vi "Next Post Processor Name.vi"(7 "Ack Result":refnum<class "Acquired Result.lvclass">, 8 "error in (no error)":errorcluster, 11 "Monitor-Pulse in":refnum<class "Batch Processor.lvclass">) -> (0 "error out":errorcluster, 1 "Complete":bool, 2 "Post processor name":string, 3 "Monitor-Pulse out":refnum<class "Batch Processor.lvclass">, 5 "Ack Result out":refnum<class "Acquired Result.lvclass">)   [LabVIEW 2020, in "Batch Processor.lvclass"]
uses:
  Batch Processor.lvclass
  C:/GitHub/LabActor/Worker/Worker.lvclass
  C:/Program Files/National Instruments/LabVIEW 2020/vi.lib/ActorFramework/Actor/Actor.lvclass
  C:/GitHub/LabActor/Template Module/Template Module.lvclass
  NHMFL_Core/Libraries/Instruments/Results/Acquired Result/Acquired Result.lvclass
  Worker/Worker.lvclass/Worker.ctl
  <vilib>/ActorFramework/Actor/Actor.lvclass/Actor.ctl
  <vilib>/ActorFramework/Message Enqueuer/Message Enqueuer.lvclass/Message Enqueuer.ctl
  Process Controller Messages/Update Plots Msg/Update Plots Msg.lvclass/Update Plots Msg.ctl
  NHMFL_Core/Libraries/Instruments/Instrument Driver/Worker State.ctl
  Batch Processor.lvclass/Batch Processor.ctl
  Template Module/Template Module.lvclass/Template Module.ctl
  NHMFL_Core/Libraries/Instruments/Results/File Path Result/File Path Result.lvclass
  C:/GitHub/NHMFL_Core/Libraries/Instruments/Results/Acquired Result/Acquired Result.lvclass
  Template Module/Read Logger.vi
  Template Module/Write Logger.vi
  Template Module/Write State.vi
  Template Module/Read State.vi
  Worker/Read File Path.vi
  <vilib>/ActorFramework/Message Enqueuer/Init from Existing Queue.vi
  <vilib>/ActorFramework/Message Enqueuer/Enqueue.vi
  Process Controller Messages/Update Plots Msg/Update Plots Msg.lvclass
  C:/Program Files/National Instruments/LabVIEW 2020/vi.lib/ActorFramework/Message/Message.lvclass
  <vilib>/ActorFramework/Message Priority Queue/Priority Enqueue.vi
  <vilib>/ActorFramework/Message Enqueuer/Message Enqueuer.lvclass
  Loggers/Logger/Logger.lvclass
  Application Controller/Application Controller.lvclass
  <vilib>/ActorFramework/Actor/Actor.lvclass
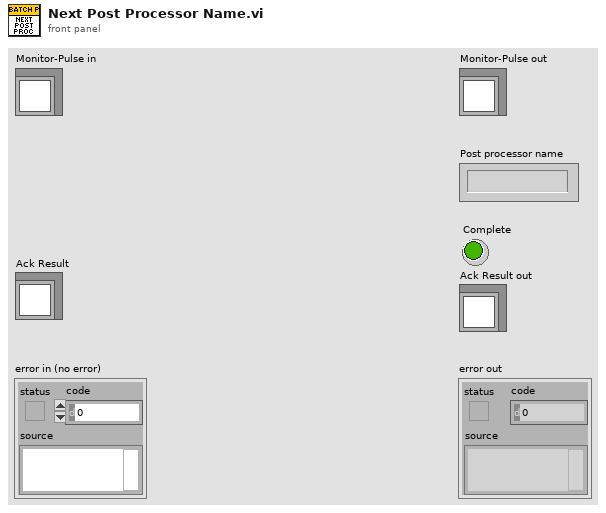
[diagram p1: front panel]
types:
  T1 = typedef "Worker State.ctl" = enum16{"Idle", "Starting", "Working", "Stopping"}
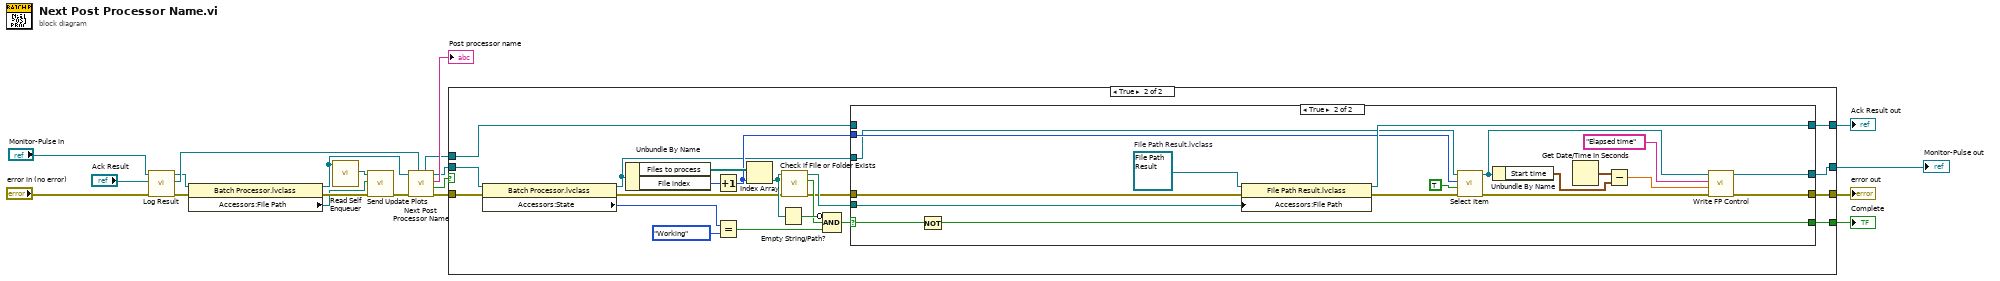
[diagram p0: block diagram]
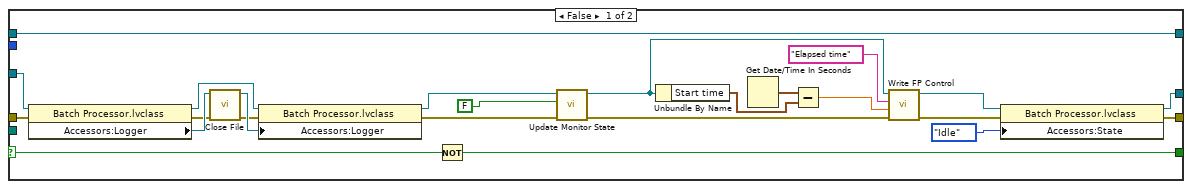
[diagram p3: hidden frame]
diagram:
  n1 = call-dynamic "Log Result.vi"("error in (no error)"="error in (no error)", "Result"="Ack Result", "Process Controller in"="Monitor-Pulse in") -> ("error out"=w9:errorcluster, "Result out"=w3:refnum<class "Acquired Result.lvclass">, "Process Controller out"=w2:refnum<class "Batch Processor.lvclass">)  [unwired: 6 in]
  n2 = property class="Batch Processor.lvclass"(reference=w2, error in=w9) -> (reference out=w1:refnum<class "Batch Processor.lvclass">, error out=w6:errorcluster, "Accessors:File Path"=w4:path)
  n3 = call <vilib>:"Read Self Enqueuer.vi"("Actor"=w1) -> ("Self Enqueuer"=w7:refnum<class "Message Enqueuer.lvclass">)  [unwired: 10 in]
  n4 = call "Send Update Plots.vi"("error in (no error)"=w6, "File Path"=w4, "Message Enqueuer"=w7) -> ("error out"=w5:errorcluster)  [unwired: 7 in, 1 out]
  n5 = call-parent "Next Post Processor Name.vi"("Ack Result"=w3, "error in (no error)"=w5, "Application Controller in"=w1) -> ("error out"=w19:errorcluster, "Complete"=w17:bool, "Post processor name"=→"Post processor name":string, "Application Controller out"=w18:refnum<class "Batch Processor.lvclass">, "Ack Result out"=w8:refnum<class "Acquired Result.lvclass">)  [unwired: 4 in]
  n6 = case shown="True" w17 {
    selector: w17 -> [w21 _]
    tunnel: w18 -> [w23 w32]
    tunnel: w19 -> [w24 w30]
    tunnel: [w24 w37] -> w15
    tunnel: [w23 w36] -> w16
    tunnel: w8 -> [w22 w33]
    tunnel: [w22 w35] -> w14
    tunnel: [w21 w34] -> w13
    frame False {
    }
    frame True {
      n7 = property class="Batch Processor.lvclass"(reference=w32, error in=w30) -> (reference out=w31:refnum<class "Batch Processor.lvclass">, error out=w29:errorcluster, "Accessors:State"=w28:T1)
      n8 = Unbundle By Name(w31) -> ("Files to process"=w45:path[], "File index"=w39:i32)
      n9 = Increment(x=w39) -> (x+1=w38:i32)
      n10 = Equal?(x=w28, y=Worker_State."Working") -> (x = y?=w26:bool)
      n11 = Index Array(array=w45, index=w38) -> (element=w44:path)
      n12 = Empty String/Path?(string/path=w44) -> (empty?=w43:bool)
      n13 = call <vilib>:"Check if File or Folder Exists.vi"("error in (no error)"=w29, "path"=w44) -> ("error out"=w40:errorcluster, "file or folder exists?"=w42:bool, "dup path"=w41:path)  [unwired: 7 in]
      n14 = Compound Arithmetic op=AND(invert w43, w42, w26) -> (w25:bool)
      n15 = case shown="True" w25 {
        selector: w25 -> [w65 w84]
        tunnel: w31 -> [w69 w71]
        tunnel: w41 -> [_ w87]
        tunnel: w40 -> [w68 w86]
        tunnel: w38 -> [_ w80]
        tunnel: [w56 w73] -> w37
        tunnel: [w54 w72] -> w36
        tunnel: [w63 w85] -> w35
        tunnel: [w64 w83] -> w34
        tunnel: w33 -> [w63 _]
        frame False {
          n16 = property class="Batch Processor.lvclass"(reference=w69, error in=w68) -> (reference out=w50:refnum<class "Batch Processor.lvclass">, error out=w51:errorcluster, "Accessors:Logger"=w52:refnum<class "Logger.lvclass">)
          n17 = call-dynamic "Close File.vi"("error in (no error)"=w51, "Logger in"=w52) -> ("error out"=w48:errorcluster, "Logger out"=w49:refnum<class "Logger.lvclass">)  [unwired: 6 in, 2 out]
          n18 = property class="Batch Processor.lvclass"(reference=w50, error in=w48, "Accessors:Logger"=w49) -> (reference out=w47:refnum<class "Batch Processor.lvclass">, error out=w46:errorcluster)
          n19 = Not(x=w65) -> (.not. x?=w64:bool)
          n20 = call-dynamic "Update Monitor State.vi"("error in (no error)"=w46, "Monitor Running"=FALSE, "Application Controller in"=w47) -> ("error out"=w66:errorcluster, "Application Controller out"=w60:refnum<class "Batch Processor.lvclass">)  [unwired: 7 in]
          n21 = Unbundle By Name(w60) -> ("Start time"=w58:timestamp)
          n22 = Get Date/Time In Seconds() -> (seconds since 1Jan1904=w59:timestamp)
          n23 = Subtract(x=w59, y=w58) -> (x-y=w57:dbl)
          n24 = call-dynamic "Write FP Control.vi"("error in (no error)"=w66, "Control Value"=w57, "Control Name"="Elapsed time", "Measure Object in"=w60) -> ("error out"=w62:errorcluster, "Measure Object out"=w55:refnum<class "Batch Processor.lvclass">)  [unwired: 6 in]
          n25 = property class="Batch Processor.lvclass"(reference=w55, error in=w62, "Accessors:State"=Worker_State."Idle" ("State")) -> (reference out=w54:refnum<class "Batch Processor.lvclass">, error out=w56:errorcluster)
        }
        frame True {
          w82 = refnum<class "File Path Result.lvclass"> refnum  # File Path Result.lvclass
          n26 = Not(x=w84) -> (.not. x?=w83:bool)
          n27 = property class="File Path Result.lvclass"(reference=w82, error in=w86, "Accessors:File Path"=w87) -> (reference out=w85:refnum<class "File Path Result.lvclass">, error out=w81:errorcluster)
          n28 = call-dynamic "Select Item.vi"("error in (no error)"=w81, "Update internal index"=TRUE, "Item index"=w80, "Batch Processor in"=w71) -> ("error out"=w74:errorcluster, "Batch Processor out"=w70:refnum<class "Batch Processor.lvclass">)  [unwired: 6 in]
          n29 = Unbundle By Name(w70) -> ("Start time"=w76:timestamp)
          n30 = Get Date/Time In Seconds() -> (seconds since 1Jan1904=w77:timestamp)
          n31 = Subtract(x=w77, y=w76) -> (x-y=w75:dbl)
          n32 = call-dynamic "Write FP Control.vi"("error in (no error)"=w74, "Control Value"=w75, "Control Name"="Elapsed time", "Measure Object in"=w70) -> ("error out"=w73:errorcluster, "Measure Object out"=w72:refnum<class "Batch Processor.lvclass">)  [unwired: 6 in]
        }
      }
    }
  }
  "error out" <- w15
  "Monitor-Pulse out" <- w16
  "Complete" <- w13
  "Ack Result out" <- w14
